vi "ClearPatterns.vi"(8 "Error In":errorcluster {"code" format="%.0x"}, 11 "Cards In":cluster{"Session":u32, "Card number":u32}[](array[cluster])) -> (0 "Error Out":errorcluster, 3 "Cards Out":cluster{"Session":u32, "Card number":u32}[](array[cluster]))   [LabVIEW 2012, in "Virtual-PGA.lvlib"]
doc: "This VI clears the pattern from the hardware, i.e. opens all relays."
uses:
  Virtual-PGA.lvlib
  Controls/Pattern.ctl
  Controls/Input.ctl
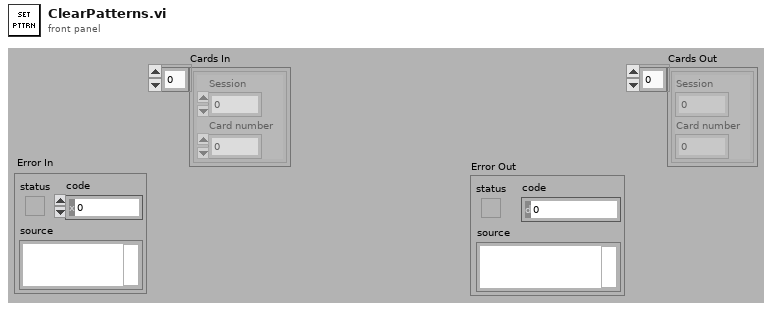
[diagram p1: front panel]
types:
  T1 = typedef "Virtual-PGA.lvlib/Pattern.ctl" = cluster{"Name":string, "Description":string, "Inputs":T2[]}
  T2 = typedef "Virtual-PGA.lvlib/Input.ctl" = cluster{"ID":string, "Label":string, "Pads":u32[]}
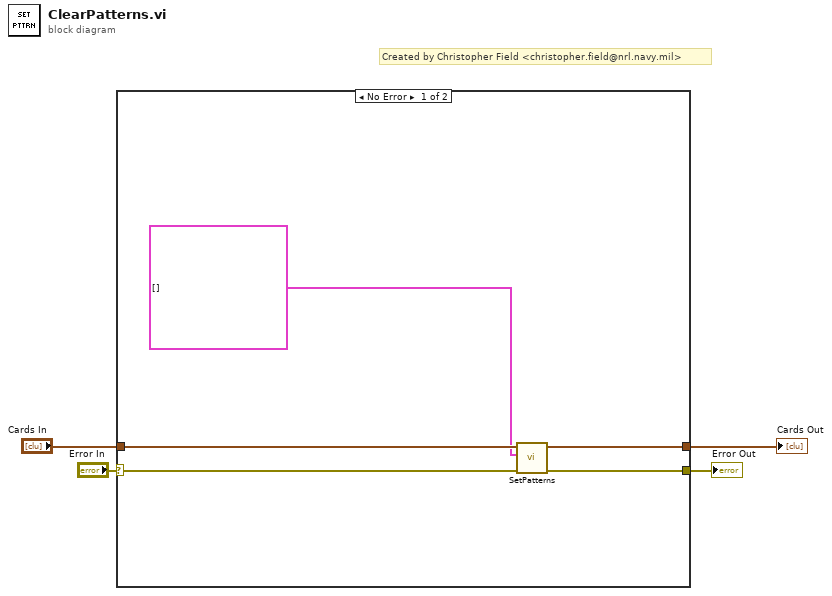
[diagram p0: block diagram]
diagram:
  # "Created by Christopher Field <christopher.field@nrl.navy.mil>"
  n1 = case shown="No Error" "Error In" {
    selector: "Error In" -> [w6 w10]
    tunnel: [w9 w10] -> w4
    tunnel: "Cards In" -> [w8 w11]
    tunnel: [w7 w11] -> w2
    frame No Error {
      n2 = call "SetPatterns.vi"("Error In"=w6, "Patterns"=T1[] [], "Cards In"=w8) -> ("Error Out"=w9:errorcluster, "Cards Out"=w7:cluster{"Session":u32, "Card number":u32}[])  [unwired: 7 in]
    }
    frame Error {
    }
  }
  "Error Out" <- w4
  "Cards Out" <- w2
